vi "chaos crest cu get.vi"(7 "maxsize":i32, 9 "output":string, 10 "cuname":string, 11 "h":u32) -> (1 "output out":string, 2 "function return":u32, 3 "h out":u32)   [LabVIEW 2014, in "libcommon-crest.lvlib"]
doc: "uint64_t chaos_crest_cu_get(chaos_crest_handle_t h,const char*cuname,char*output,int maxsize);"
uses:
  libcommon-crest.lvlib
  chaos-i686-dynamic-release/lib/libcommon-crest.so
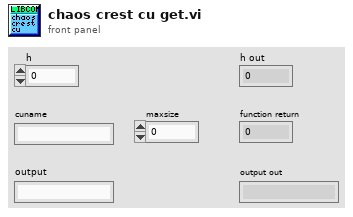
[diagram p1: front panel]
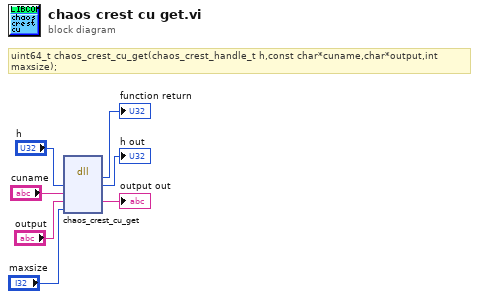
[diagram p0: block diagram]
diagram:
  # "uint64_t chaos_crest_cu_get(chaos_crest_handle_t h,const char*cuname,char*output,int maxsize);"
  n1 = dll-call lib="home/chaos/chaos_bundle/chaos-i686-dynamic-release/lib/libcommon-crest.*" fn="chaos_crest_cu_get"("h"="h", "cuname"="cuname", "output"="output", "maxsize"="maxsize") -> (→"function return":u32, "h"=→"h out":u32, "output"=→"output out":string)  [unwired: 5 in, 2 out]
